vi "Day02-04_SubVI 테스트.vi"() -> ()   [LabVIEW 2021]
panel:
  out "출력결과":dbl
  out "x+y":dbl
  in  "숫자형 4":dbl
  in  "숫자형 3":dbl
  in  "숫자형 2":dbl
  in  "숫자형":dbl
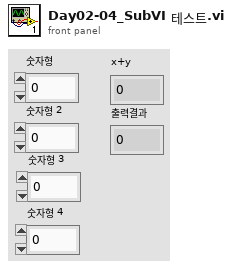
[diagram p1: front panel]
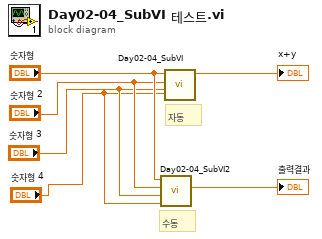
[diagram p0: block diagram]
diagram:
  # "수동"
  # "자동"
  n1 = call "Day02-04_SubVI2.vi"("더하기 4"="숫자형 4", "빼기 3"="숫자형 3", "더하기 2"="숫자형 2", "더하기1"="숫자형") -> ("출력결과"=→"출력결과":dbl)  [unwired: 7 in]
  n2 = call "Day02-04_SubVI.vi"("숫자형 4"="숫자형 4", "숫자형 3"="숫자형 3", "숫자형 2"="숫자형 2", "숫자형"="숫자형") -> ("x+y"=→"x+y":dbl)  [unwired: 7 in]
